vi "LOOP LED.vi"(8 "error in (no error)":errorcluster) -> (0 "error out":errorcluster)   [LabVIEW 2023]
uses:
  Global INIT.vi
  <vilib>/Rock Robotics/Network Tables/NT Write Integer.vi
panel:
  in  "String":string="1 - Rainbow, Rainbow Palette\n2 - Rainbow, Party Palette\n3 - Rainbow, Ocean Palette\n4 - Rainbow, Lave Palette\n5 - Rainbow, Forest Palette\n6 - Rainbow with Glitter\n7 - Confetti\n8 - Shot, Red\n9 - Shot, Blue\n10 - Shot, White\n11 - Sinelon, Rainbow Palette\n12 - Sinelon, Party Palette\n13 - Sinelon, Ocean Palette\n14 - Sinelon, Lava Palette\n15 - Sinelon, Forest Palette\n16 - Beats per Minute, Rainbow Palette\n17 - Beats per Minute, Party Palette\n18 - Beats per Minute, Ocean Palette\n19 - Beats per Minute, Lava Palette\n20 - Beats per Minute, Forest Palette\n21 - Fire, Medium\n22 - Fire, Large\n23 - Twinkles, Rainbow Palette\n24 - Twinkles, Party Palette\n25 - Twinkles, Ocean Palette\n26 - Twinkles, Lava Palette\n27 - Twinkles, Forest Palette\n28 - Color Waves, Rainbow Palette\n29 - Color Waves, Party Palette\n30 - Color Waves, Ocean Palette\n31 - Color Waves, Lava Palette\n32 - Color Waves, Forest Palette\n33 - Larson Scanner, Red\n34 - Larson Scanner, Gray\n35 - Light Chase, Red\n36 - Light Chase, Blue\n37 - Light Chase, Gray\n38 - Heartbeat, Red\n39 - Heartbeat, Blue\n40 - Heartbeat, White\n41 - Heartbeat, Gray\n42 - Breath, Red\n43 - Breath, Blue\n44 - Breath, Gray\n45 - Strobe, Red\n46 - Strobe, Blue\n47 - Strobe, Gold\n48 - Strobe, White\n49 - Color 1: End to End Blend to Black\n50 - Color 1: Larson Scanner\n51 - Color 1: Light Chase\n52 - Color 1: Heartbeat Slow\n53 - Color 1: Heartbeat Medium\n54 - Color 1: Heartbeat Fast\n55 - Color 1: Breath Slow\n56 - Color 1: Breath Fast\n57 - Color 1: Shot\n58 - Color 1: Strobe\n59 - Color 2: End to End Blend to Black\n60 - Color 2: Larson Scanner\n61 - Color 2: Light Chase\n62 - Color 2: Heartbeat Slow\n63 - Color 2: Heartbeat Medium\n64 - Color 2: Heartbeat Fast\n65 - Color 2: Breath Slow\n66 - Color 2: Breath Fast\n67 - Color 2: Shot\n68 - Color 2: Strobe\n69 - Color 1/2: Sparkle, Color 1 on Color 2\n70 - Color 1/2: Sparkle, Color 2 on Color 1\n71 - Color 1/2: Color Gradient, Color 1 and 2\n72 - Color 1/2: Beats per Minute, Color 1 and 2\n73 - Color 1/2: End to End Blend, Color 1 to 2\n74 - Color 1/2: End to End Blend\n75 - Color 1/2:  no blending (Setup Pattern)\n76 - Color 1/2: Twinkles\n77 - Color 1/2: Color Waves\n78 - Color 1/2: Sinelon\n79 - Solid Hot Pink\n80 - Solid Dark red\n81 - Solid Red\n82 - Solid Red Orange\n83 - Solid Orange\n84 - Solid Gold\n85 - Solid Yellow\n86 - Solid Lawn Green\n87 - Solid Lime\n88 - Solid Dark Green\n89 - Solid Green\n90 - Solid Blue Green\n91 - Solid Aqua\n92 - Solid Sky Blue\n93 - Solid Dark Blue\n94 - Solid Blue\n95 - Solid Blue Violet\n96 - Solid Violet\n97 - Solid White\n98 - Solid Gray\n99 - Solid Dark Gray\n100 - Solid Black\n"
  out "stack name":string
  out "pattern\nindex":u16
  out "PULSE value":dbl
  out "SPARK\nvalue":dbl
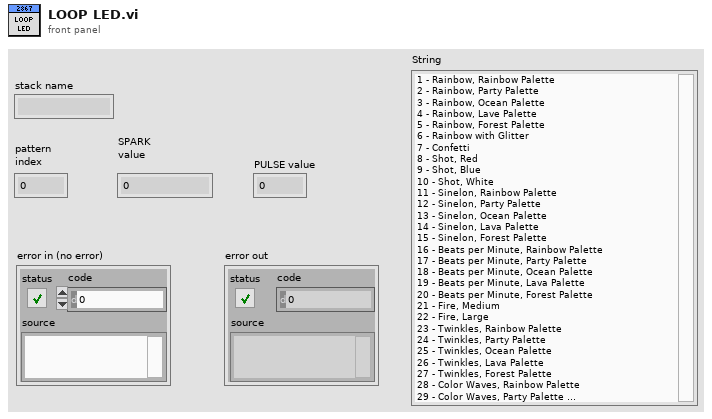
[diagram p1: front panel]
types:
  T1 = typedef "ctrl LED init.ctl" = cluster{"PWM Channel":T2, "refnum name":string, "initial output":dbl, "stack name":string, "Installed?":bool, "pattern":T3}
  T2 = typedef "FPGA_DIOPWMChannel.ctl" = enum8{"PWM 0", "PWM 1", "PWM 2", "PWM 3", "PWM 4", "PWM 5", "PWM 6", "PWM 7", "PWM 8", "PWM 9", "PWM MXP 0", "PWM MXP 1", "PWM MXP 2", "PWM MXP 3", "PWM MXP 4", "PWM MXP 5", "PWM MXP 6", "PWM MXP 7", "PWM MXP 8", "PWM MXP 9", "Invalid"}
  T3 = typedef "ctrl LED PATTERNS.ctl" = u16
  T4 = typedef "WPI_MotorControlDeviceRef.ctl" = cluster{"DeviceStatus":errorcluster, "Type":T5, "PWM":cluster{"PWM Channel":T2, "DeadBand":T6}, "CAN":cluster{"Device Number":u8, "SetOutput VI Ref":variant, "GetOutput VI Ref":variant, "Enable VI Ref":variant, "Disable VI Ref":variant, "Data":variant}, "Invert":bool, "DIO PWM":cluster{"PWM \"Enable\" Channel":T2, "DIOChannel":T7, "PWM Rate":dbl}}
  T5 = typedef "WPI_MotorControlType.ctl" = enum16{"PWM", "CAN", "DIO PWM"}
  T6 = typedef "WPI_PWMDeadband.ctl" = cluster{"Name":string, "maxPositivePwm":i32, "minPositivePwm":i32, "centerPwm":i32, "maxNegativePwm":i32, "minNegativePwm":i32, "angularRange":u16}
  T7 = typedef "FPGA_DIOChannel.ctl" = enum8{"DIO 0", "DIO 1", "DIO 2", "DIO 3", "DIO 4", "DIO 5", "DIO 6", "DIO 7", "DIO 8", "DIO 9", "DIO MXP 0", "DIO MXP 1", "DIO MXP 2", "DIO MXP 3", "DIO MXP 4", "DIO MXP 5", "DIO MXP 6", "DIO MXP 7", "DIO MXP 8", "DIO MXP 9", "DIO MXP 10", "DIO MXP 11", "DIO MXP 12", "DIO MXP 13", "DIO MXP 14", "DIO MXP 15", "SPI Port CS1", "SPI Port CS2", "SPI Port CS3", "SPI Port MISO", "SPI Port MOSI", "Invalid"}
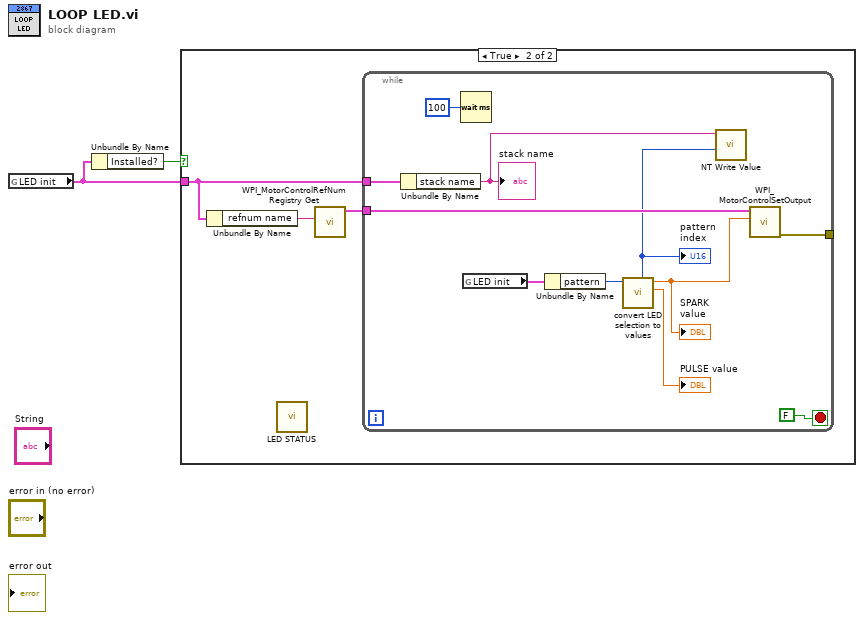
[diagram p0: block diagram]
diagram:
  n1 = global read "Global INIT.vi" "LED init"() -> (w2:T1)
  n2 = Unbundle By Name(w2) -> ("Installed?"=w1:bool)
  n3 = case shown="True" w1 {
    tunnel: w2 -> [_ w3]
    frame False {
    }
    frame True {
      n4 = Unbundle By Name(w3) -> ("refnum name"=w5:string)
      n5 = call "LED STATUS.vi"() -> ()  [unwired: 12 in]
      n6 = call <vilib>:"WPI_MotorControlRefNum Registry Get.vi"("refnum name"=w5) -> ("MotorControlDevRef"=w4:T4)  [unwired: 9 in, 1 out]
      n7 = while {
        tunnel: w4 -> [w13]
        tunnel: w3 -> [w15]
        tunnel: [w10] -> _
        stop <- FALSE stop-if-true
        n8 = Unbundle By Name(w15) -> ("stack name"=w6:string)
        "stack name" <- w6
        n9 = Wait (ms)(milliseconds to wait=u32 100) -> ()  [unwired: 1 out]
        n10 = global read "Global INIT.vi" "LED init"() -> (w12:T1)
        n11 = Unbundle By Name(w12) -> ("pattern"=w11:T3)
        n12 = call "convert LED selection to values.vi"("Blinkin LED pattern"=w11) -> ("PULSE value"=→"PULSE value":dbl, "SPARK value"=w8:dbl, "pattern\nindex"=w9:u16)  [unwired: 8 in]
        "SPARK\nvalue" <- w8
        "pattern\nindex" <- w9
        n13 = call-poly <vilib>:"NT Write Value.vi"("value"=w9, "name"=w6) -> ()  [unwired: 9 in, 1 out]
        n14 = call <vilib>:"WPI_MotorControlSetOutput.vi"("Output"=w8, "MotorControlDevRef"=w13) -> ("error out"=w10:errorcluster)  [unwired: 7 in, 2 out]
      }
    }
  }
